vi "PCE_answer_poly.vi"   [LabVIEW 2010]
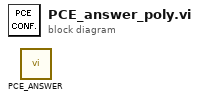
[diagram p0: block diagram]
diagram:
  n1 = call "PCE_ANSWER.vi"() -> ()  [unwired: 2 in]
